vi "Get Channels per Device.vi"(8 "error in (no error)":errorcluster, 11 "RIO Target in":refnum<class "RIO Target.lvclass">) -> (0 "error out":errorcluster, 1 "Number of Devices":i32, 2 "Channels per Device":string[][](array[string]), 3 "RIO Target out":refnum<class "RIO Target.lvclass">, 4 "Number of Channels":u32, 5 "Number of Buses":i32)   [LabVIEW 2014, in "RIO Target.lvclass"]
uses:
  RIO Target.lvclass
  <vilib>/NI/Configuration Framework/Node/NISE_CEF_Node.lvclass/NISE_CEF_Node.ctl
  Bus/Bus.lvclass
  Device node/Device.lvclass
  Device Configuration/Device Configuration.lvclass
  Device Configuration/Device Configuration.lvclass/Device Configuration.ctl
  <vilib>/NI/Configuration Framework/Node/NISE_CEF_Node.lvclass
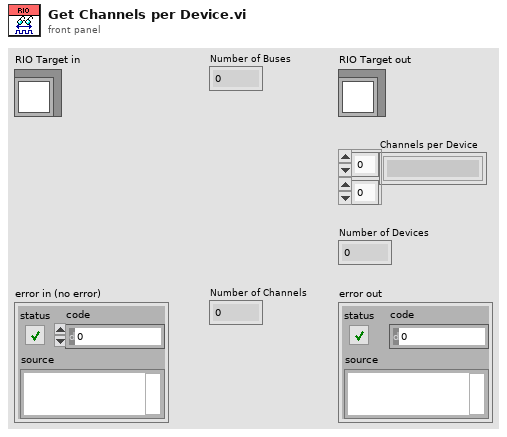
[diagram p1: front panel]
types:
  T1 = typedef "NISE_CEF_Node.lvclass/NodeRef.ctl" = refnum<data-value>
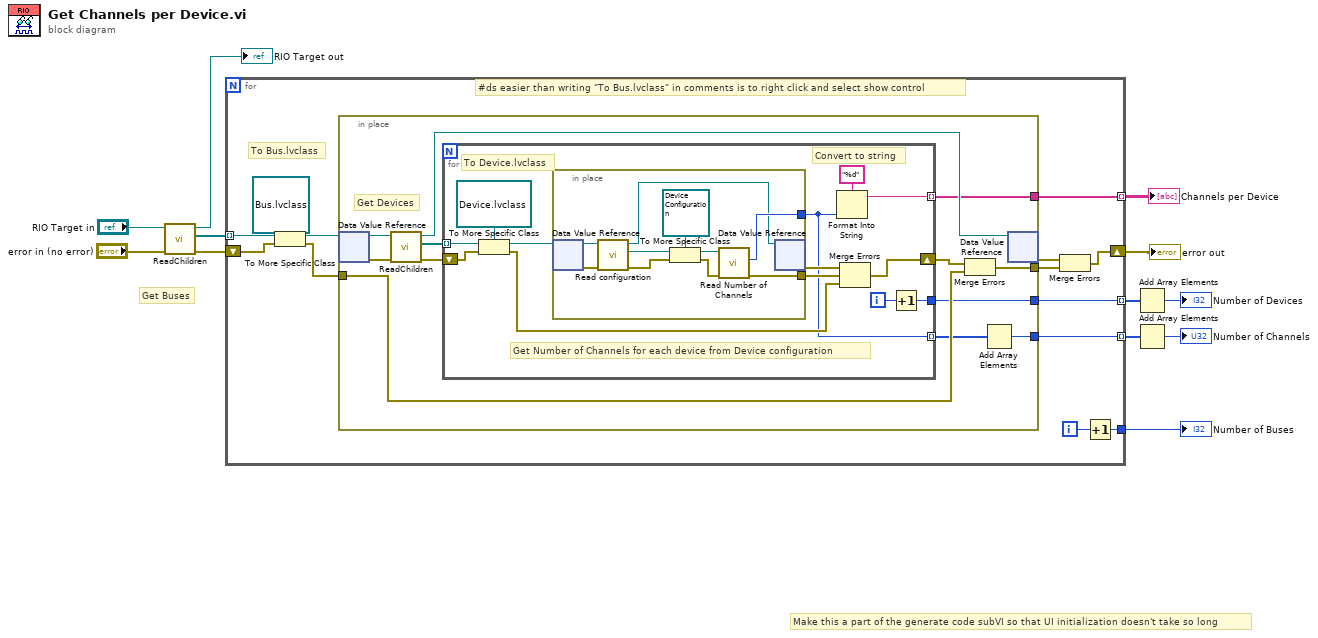
[diagram p0: block diagram]
diagram:
  # "Get Buses"
  # "Make this a part of the generate code subVI so that UI initialization doesn't take so long"
  n1 = call <vilib>:"ReadChildren.vi"("error in"="error in (no error)", "node in"="RIO Target in") -> ("error out"=w6:errorcluster, "output array"=w8:T1[], "node out"=→"RIO Target out":refnum<class "RIO Target.lvclass">)  [unwired: 7 in]
  n2 = for {
    tunnel: w8 -> [w25] mode=indexing
    tunnel: [w22] -> w12 mode=indexing
    shift-right: [w17] -> w11
    shift-left: w6 -> [w21]
    tunnel: [w16] -> w5 mode=indexing
    tunnel: [w15] -> w3 mode=indexing
    tunnel: [w13] -> w1
    i -> [w14]
    # "#ds easier than writing \"To Bus.lvclass\" in comments is to right click and select show control"
    # "To Bus.lvclass"
    n3 = To More Specific Class(target class=refnum<data-value> refnum ("data value reference"), reference=w25, error in=w21) -> (specific class reference=w23:refnum<data-value>, error out=w20:errorcluster)
    n4 = in-place {
      in-place-border: [w35] -> w22
      in-place-border: w20 -> [w30]
      in-place-border: [w29] -> w18
      in-place-border: [w27] -> w16
      in-place-border: [w26] -> w15
      # "Get Devices"
      n5 = in-place-dvr #1(w23) -> (w34:refnum<class "Bus.lvclass">, w33:errorcluster)
      n6 = call <vilib>:"ReadChildren.vi"("error in"=w33, "node in"=w34) -> ("error out"=w32:errorcluster, "output array"=w37:T1[], "node out"=w36:refnum<class "Bus.lvclass">)  [unwired: 7 in]
      n7 = for {
        tunnel: w37 -> [w50] mode=indexing
        tunnel: [w47] -> w35 mode=indexing
        shift-right: [w42] -> w31
        shift-left: w32 -> [w45]
        tunnel: [w40] -> w28 mode=indexing
        tunnel: [w38] -> w26
        i -> [w39]
        # "Convert to string"
        # "Get Number of Channels for each device from Device configuration"
        # "To Device.lvclass"
        n8 = To More Specific Class(target class=refnum<data-value> refnum ("data value reference"), reference=w50, error in=w45) -> (specific class reference=w48:refnum<data-value>, error out=w41:errorcluster)
        n9 = in-place {
          in-place-border: [w53] -> w40
          in-place-border: [w51] -> w43
          n10 = in-place-dvr #2(w48) -> (w60:refnum<class "Device.lvclass">, w56:errorcluster)
          n11 = call-dynamic "Read configuration.vi"("error in"=w56, "Device in"=w60) -> ("error out"=w55:errorcluster, "configuration"=w59:refnum<class "NISE_CEF_serializable configuration.lvclass">, "Device out"=w52:refnum<class "Device.lvclass">)  [unwired: 7 in]
          n12 = To More Specific Class(target class=refnum<class "Device Configuration.lvclass"> refnum ("Device Configuration.lvclass"), reference=w59, error in=w55) -> (specific class reference=w57:refnum<class "Device Configuration.lvclass">, error out=w54:errorcluster)
          n13 = call "Read Number of Channels.vi"("error in (no error)"=w54, "Device Configuration in"=w57) -> ("error out"=w51:errorcluster, "Number of Channels"=w53:u32)  [unwired: 7 in, 1 out]
          n14 = in-place-dvr #2(w52) -> (w44:errorcluster)  [unwired: 1 out]
        }
        n15 = Format Into String(format string="%d", w40) -> (resulting string=w47:string)  [unwired: 2 in, 1 out]
        n16 = Merge Errors(w44, w43, w41) -> (w42:errorcluster)
        n17 = Increment(x=w39) -> (x+1=w38:i32)
      }
      n18 = Merge Errors(w31, w30) -> (w29:errorcluster)
      n19 = Add Array Elements(numeric array=w28) -> (sum=w27:u32)
      n20 = in-place-dvr #1(w36) -> (w19:errorcluster)  [unwired: 1 out]
    }
    n21 = Merge Errors(w19, w18) -> (w17:errorcluster)
    n22 = Increment(x=w14) -> (x+1=w13:i32)
  }
  "Channels per Device" <- w12
  "error out" <- w11
  "Number of Buses" <- w1
  n23 = Add Array Elements(numeric array=w3) -> (sum=→"Number of Devices":i32)
  n24 = Add Array Elements(numeric array=w5) -> (sum=→"Number of Channels":u32)
